vi "SpecPage_ADAS_IO_Plugin.vi"(10 "Spec Page Interface":T1, 11 "MetaDataObj in":refnum<class "MetaDataObj.lvclass">) -> (3 "MetaDataObj out":refnum<class "MetaDataObj.lvclass">)   [LabVIEW 2020, in "ADAS_IO_Template_MDO.lvclass"]
uses:
  ADAS_IO_Template_MDO.lvclass
  <resource>/dialog/NewProjectWizard/Spec Page Interface.ctl
  <resource>/dialog/NewProjectWizard/MetaDataObj/MetaDataObj.lvclass
  C:/Program Files/National Instruments/LabVIEW 2020/resource/dialog/NewProjectWizard/MetaDataObj/MetaDataObj.lvclass
  <resource>/dialog/NewProjectWizard/MetaDataObj/MetaDataObj.lvclass/MetaDataObj.ctl
  <resource>/dialog/NewProjectWizard/MetaDataObj/Accessors/Read Overlay Pixmap.vi
  <resource>/dialog/NewProjectWizard/MetaDataObj/Accessors/Write Project Name.vi
  <resource>/dialog/NewProjectWizard/MetaDataObj/Accessors/Write Project Root.vi
  <resource>/dialog/NewProjectWizard/MetaDataObj/Accessors/Write Overlay Pixmap.vi
  <resource>/dialog/NewProjectWizard/MetaDataObj/Accessors/Write File Prefix.vi
  <resource>/dialog/NewProjectWizard/MetaDataObj/Accessors/Read Hide Prefix.vi
  <resource>/dialog/NewProjectWizard/MetaDataObj/Accessors/Read Hide Icon Overlay.vi
  <vilib>/LabVIEW Icon API/lv_icon/Classes/Icon/Icon.lvclass
  ADAS_IO_Template_MDO.lvclass/ADAS_IO_Template_MDO.ctl
  <resource>/dialog/NewProjectWizard/Icon Overlay/NI_NPW_Icon Overlay.lvlib
  <vilib>/LabVIEW Icon API/LabVIEW Icon API.lvlib
panel:
  in  "IO Plugin Name":string="MyNewModule"
  in  "IO Plugin Directory":path
  out "Modified Icon":picture
  in  "Sample Icon":picture
  out "Overlay (picture)":picture
  in  "Edit Icon Overlay":bool
  # "The following VI Packages must be installed before building an IO Plugin:\nOpenG File Library\nCaraya Unit Test Framework\n\nThis is version 2.0.0 of the IO Plugin Template."
  # "Modify VI Icons"
  # "+"
  # "="
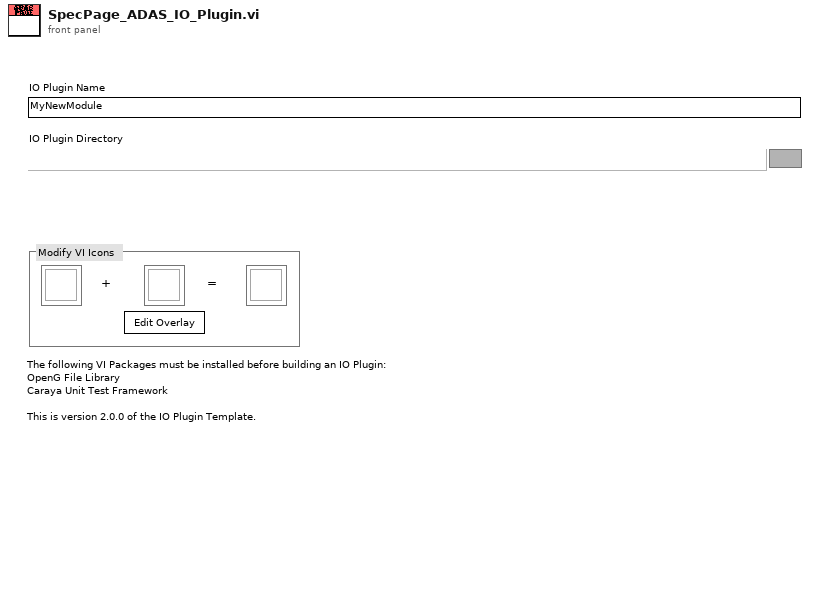
[diagram p1: front panel]
types:
  T1 = typedef "Spec Page Interface.ctl" = cluster{"\"Tab Forward To\" Refnum":refnum<vi>, "\"Tab Backward To\" Refnum":refnum<vi>, "Errors":refnum<user-event>, "Quit":refnum<user-event>}
  T2 = typedef "imagedata.ctl" = cluster{"image type":i32, "image depth":i32, "image":u8[], "mask":u8[], "colors":u32[], "Rectangle":cluster{"left":i16, "top":i16, "right":i16, "bottom":i16}}
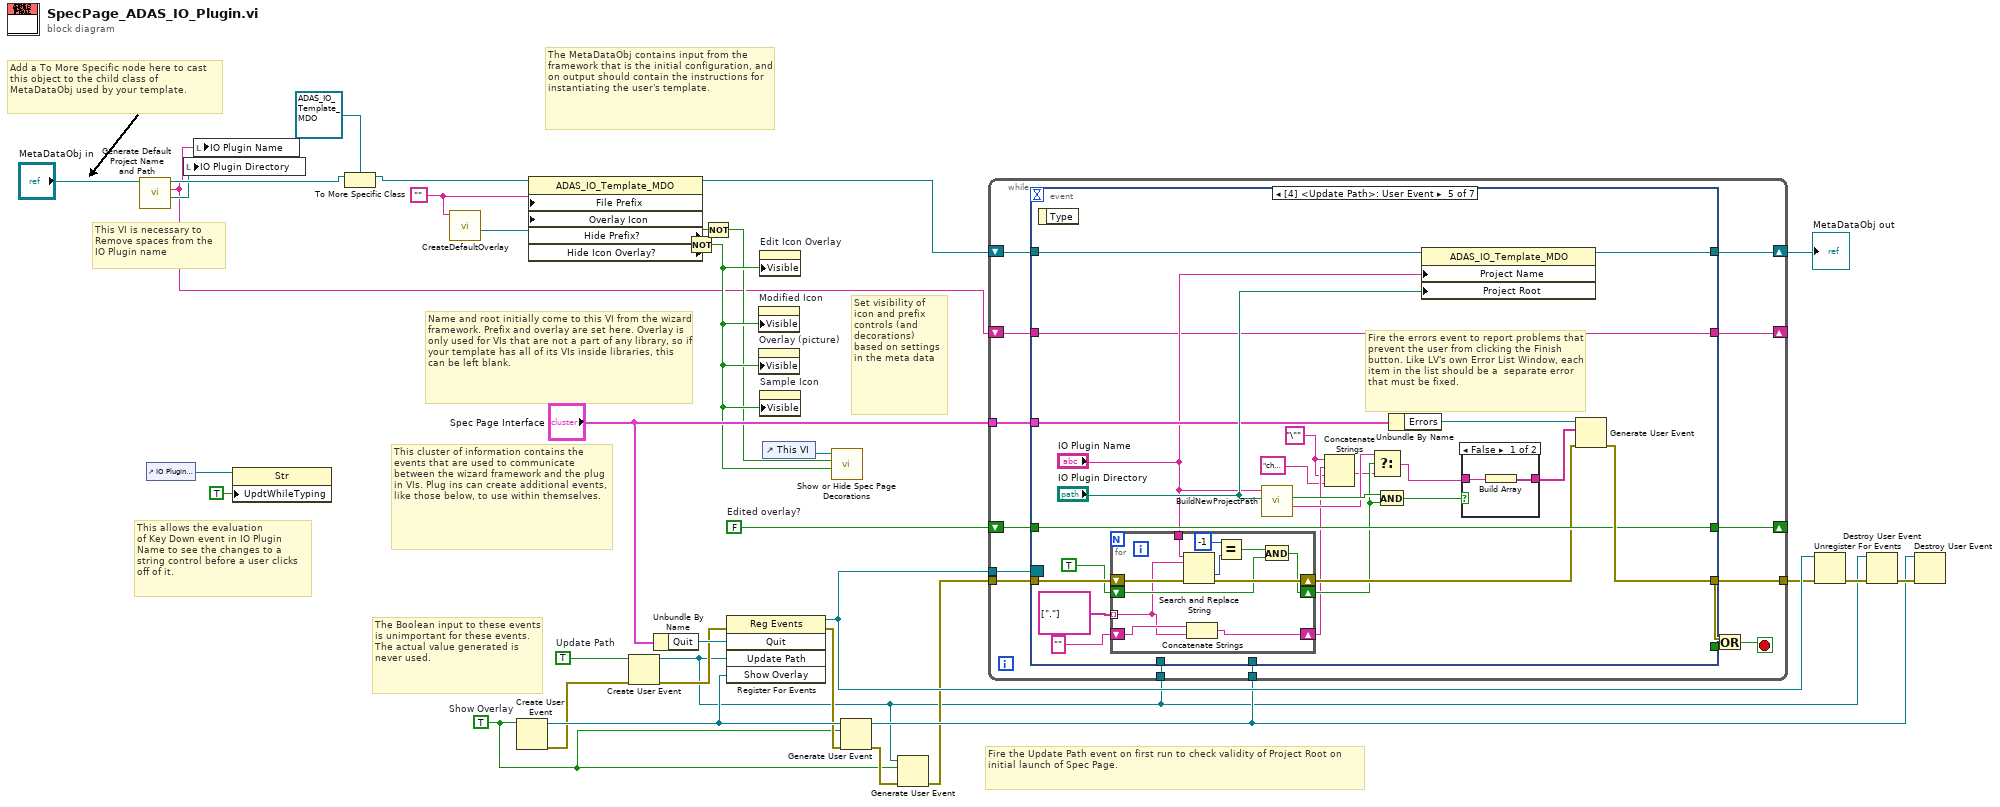
[diagram p0: block diagram]
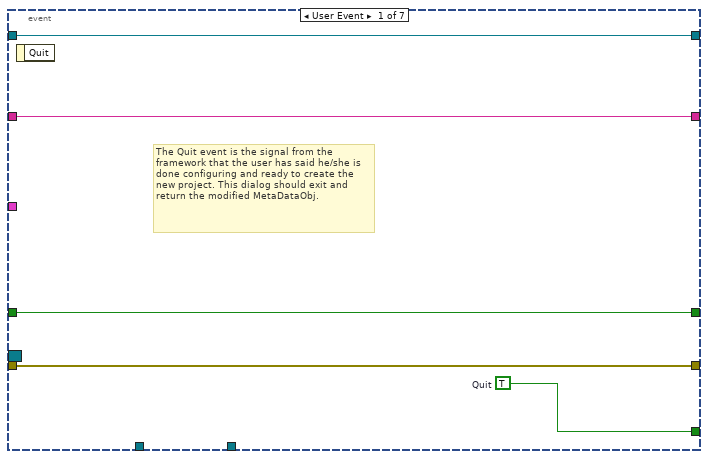
[diagram p2: hidden frame]
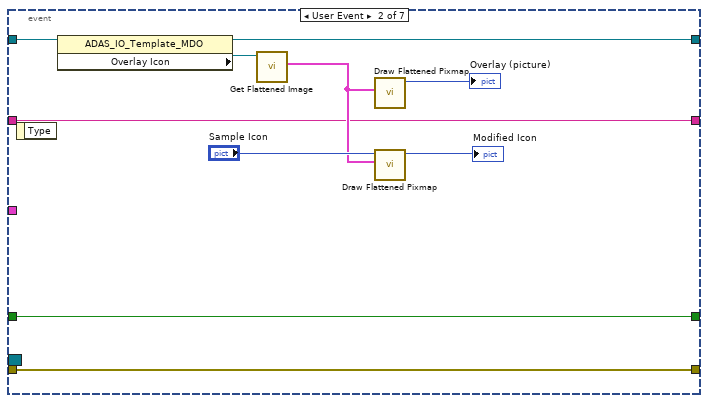
[diagram p3: hidden frame]
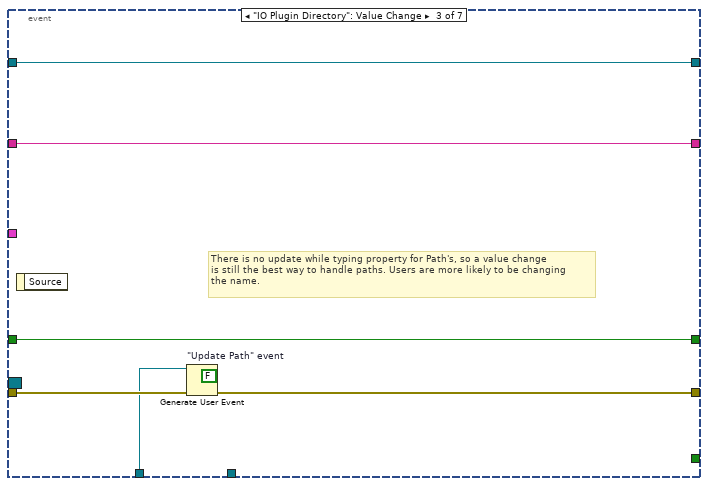
[diagram p4: hidden frame]
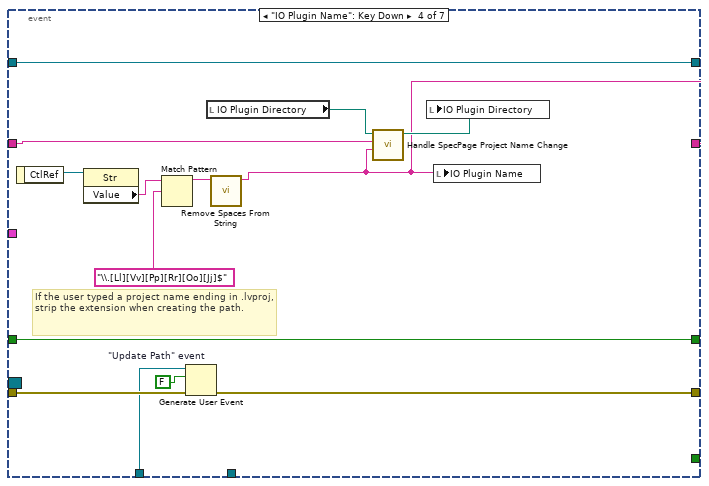
[diagram p5: hidden frame]
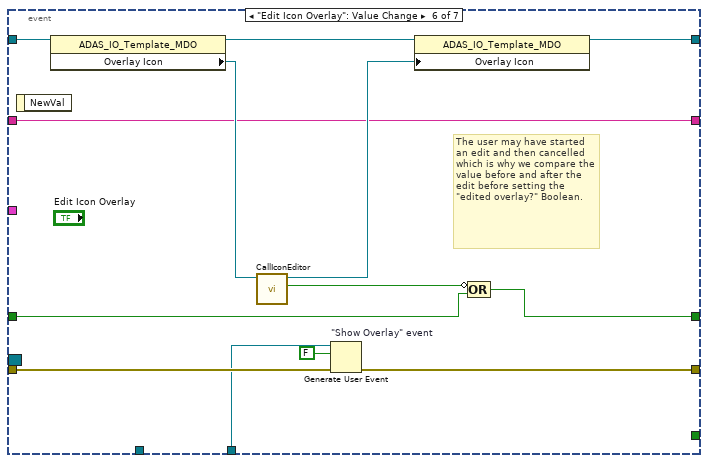
[diagram p7: hidden frame]
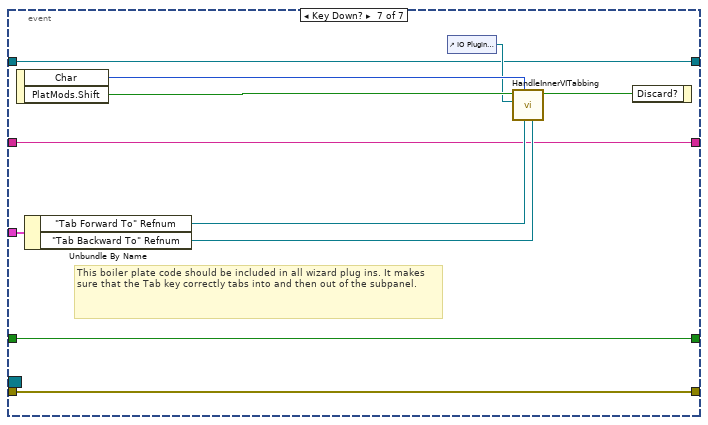
[diagram p8: hidden frame]
diagram:
  w9 = ""
  w25 = FALSE  # Edited overlay?
  w18 = TRUE  # Show Overlay
  w30 = TRUE  # Update Path
  # "This allows the evaluation\nof Key Down event in IO Plugin\nName to see the changes to a \nstring control before a user clicks\noff of it."
  # "This VI is necessary to \nRemove spaces from the\nIO Plugin name"
  # "Set visibility of icon and prefix controls (and decorations) based on settings in the meta data"
  # "Fire the Update Path event on first run to check validity of Project Root on initial launch of Spec Page."
  # "The Boolean input to these events is unimportant for these events. The actual value generated is never used."
  # "This cluster of information contains the events that are used to communicate between the wizard framework and the plug in VIs. Plug ins can create additional events, like those below, to use within themselves."
  # "The MetaDataObj contains input from the framework that is the initial configuration, and on output should contain the instructions for instantiating the user's template."
  # "Add a To More Specific node here to cast this object to the child class of MetaDataObj used by your template."
  # "Name and root initially come to this VI from the wizard framework. Prefix and overlay are set here. Overlay is only used for VIs that are not a part of any library, so if your template has all of its VIs inside libraries, this can be left blank."
  n1 = call "Generate Default Project Name and Path.vi"("DNL_MetaDataObj in"="MetaDataObj in") -> ("Project Root"=w4:path, "Project Name"=w1:string, "DNL_MetaDataObj out"=w5:refnum<class "MetaDataObj.lvclass">)  [unwired: 8 in]
  n2 = control-ref of="IO Plugin Name"() -> (w3:refnum<vi>)
  n3 = local write "IO Plugin Directory"(w4) -> ()
  n4 = local write "IO Plugin Name"(w1) -> ()
  n5 = property class="Str"(reference=w3, "UpdtWhileTyping"=TRUE ("Update While Typing?")) -> ()  [unwired: 1 in, 2 out]
  n6 = To More Specific Class(target class=refnum<class "ADAS_IO_Template_MDO.lvclass"> refnum ("ADAS_IO_Template_MDO.lvclass"), reference=w5) -> (specific class reference=w8:refnum<class "ADAS_IO_Template_MDO.lvclass">)  [unwired: 1 in, 1 out]
  n7 = call <resource>:"CreateDefaultOverlay.vi"("File Prefix"=w9) -> ("Overlay Icon"=w16:refnum<class "Icon.lvclass">)  [unwired: 8 in, 2 out]
  n8 = Create User Event(user event datatype=w18) -> (user event=w24:refnum<user-event>, error out=w21:errorcluster)  [unwired: 1 in]
  n9 = property class="ADAS_IO_Template_MDO"(reference=w8, "File Prefix"=w9, "Overlay Icon"=w16) -> (reference out=w15:refnum<class "ADAS_IO_Template_MDO.lvclass">, "Hide Prefix?"=w14:bool, "Hide Icon Overlay?"=w13:bool)  [unwired: 1 in, 1 out]
  n10 = Create User Event(user event datatype=w30, error in=w21) -> (user event=w17:refnum<user-event>, error out=w29:errorcluster)
  n11 = Unbundle By Name("Spec Page Interface") -> ("Quit"=w34:refnum<user-event>)
  n12 = Not(x=w13) -> (.not. x?=w11:bool)
  n13 = Not(x=w14) -> (.not. x?=w10:bool)
  n14 = register-events(error in=w29, w34, w17, w24) -> (reference out=w33:refnum<event-registration>, error out=w22:errorcluster)  [unwired: 1 in]
  n15 = property on="Modified Icon" class="Pict"("Visible"=w11) -> ()  [unwired: 2 in, 2 out]
  n16 = property on="Overlay (picture)" class="Pict"("Visible"=w11) -> ()  [unwired: 2 in, 2 out]
  n17 = property on="Edit Icon Overlay" class="Bool"("Visible"=w11) -> ()  [unwired: 2 in, 2 out]
  n18 = property on="Sample Icon" class="Pict"("Visible"=w11) -> ()  [unwired: 2 in, 2 out]
  n19 = control-ref of="This VI"() -> (w12:refnum<vi>)
  n20 = call <resource>:"Show or Hide Spec Page Decorations.vi"("Icon Visible"=w11, "Prefix Visible"=w10, "Spec Page refnum"=w12) -> ()  [unwired: 9 in]
  n21 = Generate User Event(user event=w24, event data cluster=w18, error in=w22) -> (user event out=w23:refnum<user-event>, error out=w20:errorcluster)  [unwired: 1 in]
  n22 = Generate User Event ("\"Update Path\" event")(user event=w17, event data cluster=w18, error in=w20) -> (error out=w19:errorcluster)  [unwired: 1 in, 1 out]
  n23 = while {
    tunnel: "Spec Page Interface" -> [w46]
    shift-right: [w45] -> w27
    shift-left: w15 -> [w44]
    tunnel: w33 -> [w48]
    tunnel: w19 -> [w47]
    tunnel: [w41] -> w31
    tunnel: w17 -> [w40]
    tunnel: w23 -> [w39]
    shift-right: [w37] -> _
    shift-left: w25 -> [w38]
    shift-right: [w36] -> _
    shift-left: w1 -> [w35]
    stop <- w43 stop-if-true
    n24 = event shown="[4] <Update Path>: User Event" {
      selector: w48 -> [_ _ _ _ _ _ _]
      dyn-events: _ -> [_ _ _ _ _ _ _]
      timeout: _ -> [_ _ _ _ _ _ _]
      tunnel: w46 -> [_ _ _ _ w105 _ w141]
      tunnel: [w53 _ _ _ _ _ _] -> w42
      tunnel: [w52 w63 w69 w74 w104 w129 w135] -> w41
      tunnel: w47 -> [w52 w63 w70 w75 w100 w130 w135]
      tunnel: [w51 w58 w65 w80 w103 w134 w138] -> w45
      tunnel: w44 -> [w51 w59 w65 w80 w94 w133 w138]
      tunnel: w40 -> [_ _ w68 w73 _ _ _]
      tunnel: w39 -> [_ _ _ _ _ w128 _]
      tunnel: w38 -> [w50 w57 w66 w82 w102 w127 w137]
      tunnel: [w50 w57 w66 w82 w102 w126 w137] -> w37
      tunnel: [w49 w54 w64 w72 w93 w122 w136] -> w36
      tunnel: w35 -> [w49 w54 w64 w76 w93 w122 w136]
      event User Event {
        w53 = TRUE  # Quit
        # "The Quit event is the signal from the framework that the user has said he/she is done configuring and ready to create the new project. This dialog should exit and return the modified MetaDataObj."
        n25 = event-data() -> ()  [unwired: 1 in, 1 out]
      }
      event User Event {
        n26 = event-data() -> ()  [unwired: 1 in, 1 out]
        n27 = property class="ADAS_IO_Template_MDO"(reference=w59) -> (reference out=w58:refnum<class "ADAS_IO_Template_MDO.lvclass">, "Overlay Icon"=w56:refnum<class "Icon.lvclass">)  [unwired: 1 in, 1 out]
        n28 = call <vilib>:"Get Flattened Image.vi"("lv_icon.lvlib:Icon.lvclass in"=w56) -> ("Color Image"=w55:T2)  [unwired: 7 in, 3 out]
        n29 = call <vilib>:"Draw Flattened Pixmap.vi"("image data"=w55) -> ("new picture"=→"Overlay (picture)":picture)  [unwired: 8 in]
        n30 = call <vilib>:"Draw Flattened Pixmap.vi"("image data"=w55, "picture"="Sample Icon") -> ("new picture"=→"Modified Icon":picture)  [unwired: 7 in]
      }
      event "IO Plugin Directory": Value Change {
        # "There is no update while typing property for Path's, so a value change \nis still the best way to handle paths. Users are more likely to be changing \nthe name."
        n31 = event-data() -> ()  [unwired: 1 in, 1 out]
        n32 = Generate User Event "\"Update Path\" event"(user event=w68, event data cluster=FALSE ("event data"), error in=w70) -> (error out=w69:errorcluster)  [unwired: 1 in, 1 out]
      }
      event "IO Plugin Name": Key Down {
        # "If the user typed a project name ending in .lvproj, strip the extension when creating the path."
        n33 = event-data() -> ("CtlRef"=w78:refnum<vi>)  [unwired: 1 in]
        n34 = property class="Str"(reference=w78) -> ("Value"=w77:string)  [unwired: 1 in, 2 out]
        n35 = Match Pattern(string=w77, regular expression="\\.[Ll][Vv][Pp][Rr][Oo][Jj]$") -> (before substring=w79:string)  [unwired: 1 in, 3 out]
        n36 = Generate User Event "\"Update Path\" event"(user event=w73, event data cluster=FALSE ("event data"), error in=w75) -> (error out=w74:errorcluster)  [unwired: 1 in, 1 out]
        n37 = local read "IO Plugin Directory"() -> (w84:path)
        n38 = call "Remove Spaces From String.vi"("String in"=w79) -> ("string"=w72:string)  [unwired: 10 in]
        n39 = call <resource>:"Handle SpecPage Project Name Change.vi"("Project Name New Value"=w72, "Project Name Old Value"=w76, "Project Root in"=w84) -> ("Project Root out"=w83:path)  [unwired: 8 in]
        n40 = local write "IO Plugin Directory"(w83) -> ()
        n41 = local write "IO Plugin Name"(w72) -> ()
      }
      event User Event {
        w87 = "\"" ("string")
        # "Fire the errors event to report problems that prevent the user from clicking the Finish button. Like LV's own Error List Window, each item in the list should be a  separate error that must be fixed."
        n42 = event-data() -> ()  [unwired: 1 in, 1 out]
        n43 = for {
          tunnel: "IO Plugin Name" -> [w119]
          tunnel: string[] ["."] ("appended array") -> [w110] mode=indexing
          shift-right: [w117] -> w99
          shift-left: w100 -> [w118]
          shift-right: [w112] -> w91
          shift-left: TRUE ("x = y?") -> [w113]
          shift-right: [w109] -> w88
          shift-left: "" ("search string") -> [w111]
          n44 = Search and Replace String(input string=w119, search string=w110, error in=w118) -> (offset past replacement=w116:i32, error out=w117:errorcluster)  [unwired: 5 in, 2 out]
          n45 = Concatenate Strings(w111, w110) -> (w109:string)
          n46 = Equal?(x=-1, y=w116) -> (x = y?=w114:bool)
          n47 = And(x=w114, y=w113) -> (x .and. y?=w112:bool)
        }
        n48 = call <resource>:"BuildNewProjectPath.vi"("Project Root"="IO Plugin Directory", "Project Name"="IO Plugin Name") -> ("Error Message"=w95:string, "Valid?"=w96:bool)  [unwired: 7 in, 1 out]
        n49 = Concatenate Strings(w87, w88, w87, "character not allowed in IO Plugin Name" ("t")) -> (w85:string)
        n50 = Select(t=w95, s=w91, f=w85) -> (s? t:f=w98:string)
        n51 = And(x=w96, y=w91) -> (x .and. y?=w97:bool)
        n52 = Unbundle By Name(w105) -> ("Errors"=w108:refnum<user-event>)
        n53 = property class="ADAS_IO_Template_MDO"(reference=w94, "Project Name"="IO Plugin Name", "Project Root"="IO Plugin Directory") -> (reference out=w103:refnum<class "ADAS_IO_Template_MDO.lvclass">)  [unwired: 1 in, 1 out]
        n54 = case shown="False" w97 {
          tunnel: w98 -> [w121 _]
          tunnel: [w120 _] -> w106
          frame False {
            n55 = Build Array(w121) -> (w120:string[])
          }
          frame True {
          }
        }
        n56 = Generate User Event(user event=w108, event data cluster=w106, error in=w99) -> (error out=w104:errorcluster)  [unwired: 1 in, 1 out]
      }
      event "Edit Icon Overlay": Value Change {
        # "The user may have started an edit and then cancelled which is why we compare the value before and after the edit before setting the \"edited overlay?\" Boolean."
        n57 = event-data() -> ()  [unwired: 1 in, 1 out]
        n58 = property class="ADAS_IO_Template_MDO"(reference=w133) -> (reference out=w132:refnum<class "ADAS_IO_Template_MDO.lvclass">, "Overlay Icon"=w125:refnum<class "Icon.lvclass">)  [unwired: 1 in, 1 out]
        n59 = call <resource>:"CallIconEditor.vi"("Icon in"=w125) -> ("Canceled?"=w123:bool, "Icon out"=w124:refnum<class "Icon.lvclass">)  [unwired: 9 in]
        n60 = Generate User Event "\"Show Overlay\" event"(user event=w128, event data cluster=FALSE ("event data"), error in=w130) -> (error out=w129:errorcluster)  [unwired: 1 in, 1 out]
        n61 = property class="ADAS_IO_Template_MDO"(reference=w132, "Overlay Icon"=w124) -> (reference out=w134:refnum<class "ADAS_IO_Template_MDO.lvclass">)  [unwired: 1 in, 1 out]
        n62 = Compound Arithmetic op=OR(invert w123, w127) -> (w126:bool)
      }
      event Key Down? {
        # "This boiler plate code should be included in all wizard plug ins. It makes sure that the Tab key correctly tabs into and then out of the subpanel."
        n63 = event-data() -> ("Char"=w144:i16, "PlatMods.Shift"=w143:bool)  [unwired: 1 in]
        n64 = Unbundle By Name(w141) -> ("\"Tab Forward To\" Refnum"=w140:refnum<vi>, "\"Tab Backward To\" Refnum"=w139:refnum<vi>)
        n65 = control-ref of="IO Plugin Name"() -> (w142:refnum<vi>)
        n66 = call <resource>:"HandleInnerVITabbing.vi"("Tab Backward To"=w139, "Tab Forward To"=w140, "Char"=w144, "First Control"=w142, "Shift"=w143) -> ("Discard"=w145:bool)  [unwired: 6 in]
        n67 = event-data("Discard?"=w145) -> ()  [unwired: 1 in, 1 out]
      }
    }
    n68 = Or(x=w41, y=w42) -> (x .or. y?=w43:bool)
  }
  "MetaDataObj out" <- w27
  n69 = Unregister For Events(event registration refnum=w33, error in=w31) -> (error out=w28:errorcluster)
  n70 = Destroy User Event(user event=w17, error in=w28) -> (error out=w26:errorcluster)
  n71 = Destroy User Event(user event=w23, error in=w26) -> ()  [unwired: 1 out]
